vi "Plugin RT Driver VI.vi"(7 "Operation":T1, 11 "Device Reference in":T2 format="%.0x") -> (0 "Error Code":i32)   [LabVIEW 2024, in "FPGA Addon Engine.lvlib"]
uses:
  FPGA Addon Engine.lvlib
  <vilib>/NI VeriStand/Custom Device API/Custom Device Item Ref.ctl
  <vilib>/NI VeriStand/Custom Device API/Hardware Interface Driver VI Operation.ctl
  Plugin Framework/Plugin Framework.lvclass
  <vilib>/NI VeriStand/Custom Device API/Custom Device API.lvlib
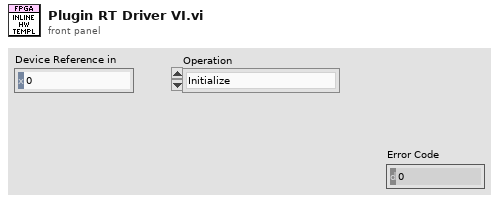
[diagram p1: front panel]
types:
  T1 = typedef "Custom Device API.lvlib/Hardware Interface Driver VI Operation.ctl" = enum16{"Initialize", "Start", "Read Data from HW", "Write Data to HW", "Close"}
  T2 = typedef "Custom Device API.lvlib/Custom Device Item Ref.ctl" = u64
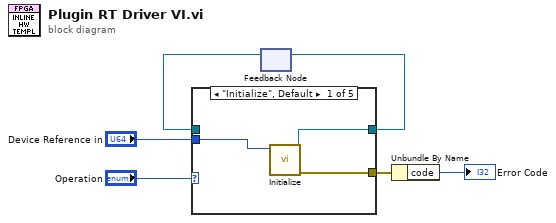
[diagram p0: block diagram]
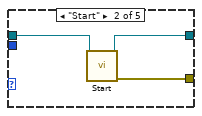
[diagram p2: hidden frame]
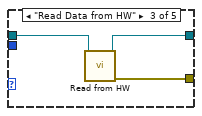
[diagram p3: hidden frame]
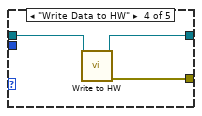
[diagram p4: hidden frame]
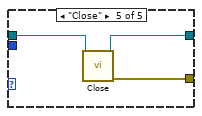
[diagram p5: hidden frame]
diagram:
  n1 = feedback #1() -> (w3:refnum<class "Plugin Framework.lvclass">)  [unwired: 1 in]
  n2 = case shown="\"Initialize\", Default" "Operation" {
    tunnel: [w8 w10 w13 w16 w19] -> w4
    tunnel: w3 -> [_ w11 w14 w17 w20]
    tunnel: "Device Reference in" -> [w7 _ _ _ _]
    tunnel: [w9 w12 w15 w18 w21] -> w6
    frame "Initialize", Default {
      n3 = call "Initialize.vi"("Custom Device Item Ref"=w7) -> ("error out"=w9:errorcluster, "Plugin Framework out"=w8:refnum<class "Plugin Framework.lvclass">)  [unwired: 9 in]
    }
    frame "Start" {
      n4 = call "Start.vi"("Plugin Framework in"=w11) -> ("error out"=w12:errorcluster, "Plugin Framework out"=w10:refnum<class "Plugin Framework.lvclass">)  [unwired: 9 in]
    }
    frame "Read Data from HW" {
      n5 = call "Read from HW.vi"("Plugin Framework in"=w14) -> ("error out"=w15:errorcluster, "Plugin Framework out"=w13:refnum<class "Plugin Framework.lvclass">)  [unwired: 9 in]
    }
    frame "Write Data to HW" {
      n6 = call "Write to HW.vi"("Plugin Framework in"=w17) -> ("error out"=w18:errorcluster, "Plugin Framework out"=w16:refnum<class "Plugin Framework.lvclass">)  [unwired: 9 in]
    }
    frame "Close" {
      n7 = call "Close.vi"("Plugin Framework in"=w20) -> ("error out"=w21:errorcluster, "Plugin Framework out"=w19:refnum<class "Plugin Framework.lvclass">)  [unwired: 9 in]
    }
  }
  n8 = feedback-in #1(w4) -> ()
  n9 = Unbundle By Name(w6) -> ("code"=→"Error Code":i32)
